vi "move stage abs.vi"(5 "blocking?":bool=TRUE, 8 "error in (no error)":errorcluster, 9 "transform cluster + actuator":T1, 10 "positions":T2, 11 "location (steps)":dbl[](array[numeric])) -> (0 "error out":errorcluster)   [LabVIEW 2015]
uses:
  pipette cleaning/pressure box/cleaning_soft/controls/actuator_type.ctl
  pipette cleaning/pressure box/cleaning_soft/controls/actuator_cluster.ctl
  machine_vision/coordinate model vis/transform_properties_actuators.ctl
  machine_vision/controls/transform_cluster_actuator.ctl
panel:
  # "move manip top lvl"
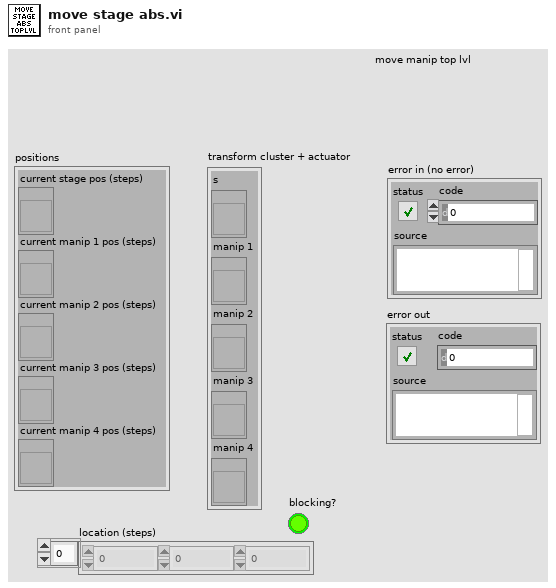
[diagram p1: front panel]
types:
  T1 = typedef "transform_cluster_actuator.ctl" = cluster{"s":refnum<vi>, "manip 1":refnum<vi>, "manip 2":refnum<vi>, "manip 3":refnum<vi>, "manip 4":refnum<vi>}
  T2 = cluster{"current stage pos (steps)":refnum<vi>, "current manip 1 pos (steps)":refnum<vi>, "current manip 2 pos (steps)":refnum<vi>, "current manip 3 pos (steps)":refnum<vi>, "current manip 4 pos (steps)":refnum<vi>}
  T3 = typedef "transform_properties_actuators.ctl" = cluster{"theta (deg)":dbl, "X sc factor (px/step)":dbl, "Y sc factor (px/step)":dbl, "zero loc (x,y,z)":dbl[], "flip y?":bool, "flip x?":bool, "gamma (deg)":dbl, "flip z?":bool, "Z sc factor (px/step)":dbl, "actuator":T4, "safe space (steps)":i32[]}
  T4 = typedef "actuator_cluster.ctl" = cluster{"Actuator COM":refnum<visa-resource-name>, "Actuator type":T5}
  T5 = typedef "actuator_type.ctl" = enum16{"Scientifica", "Sutter", "Demo", "Off"}
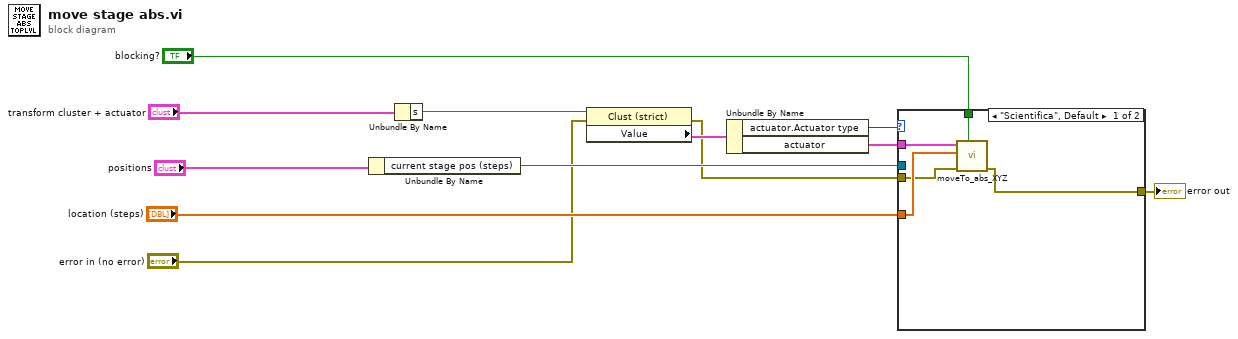
[diagram p0: block diagram]
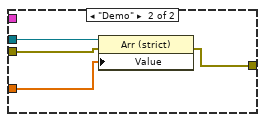
[diagram p2: hidden frame]
diagram:
  n1 = Unbundle By Name("positions") -> ("current stage pos (steps)"=w5:refnum<vi>)
  n2 = Unbundle By Name("transform cluster + actuator") -> ("s"=w9:refnum<vi>)
  n3 = property class="Clust (strict)"(reference=w9, error in="error in (no error)") -> (error out=w2:errorcluster, "Value"=w10:T3)  [unwired: 1 out]
  n4 = Unbundle By Name(w10) -> ("actuator.Actuator type"=w8:T5, "actuator"=w11:T4)
  n5 = case shown="\"Scientifica\", Default" w8 {
    tunnel: w11 -> [w17 _]
    tunnel: "blocking?" -> [w16 _]
    tunnel: w5 -> [_ w21]
    tunnel: "location (steps)" -> [w15 w20]
    tunnel: w2 -> [w14 w19]
    tunnel: [w13 w18] -> w1
    frame "Scientifica", Default {
      n6 = call "moveTo_abs_XYZ.vi"("blocking?"=w16, "error in"=w14, "XYZ location (steps)"=w15, "Actuator cluster in"=w17) -> ("error out"=w13:errorcluster)  [unwired: 6 in, 1 out]
    }
    frame "Demo" {
      n7 = property class="Arr (strict)"(reference=w21, error in=w19, "Value"=w20) -> (error out=w18:errorcluster)  [unwired: 1 out]
    }
  }
  "error out" <- w1
